vi "Test Basic Comm.vi"() -> ()   [LabVIEW 2011, in "Diamond Universal Driver.lvlib"]
uses:
  Diamond Universal Driver.lvlib
  Controls/board type.ctl
  Controls/dscBool.ctl
  Controls/dsccb.ctl
  constants.vi
  Controls/dscADSettings.ctl
  Controls/dscAIOint.ctl
  IO/DSCS.ctl
  Controls/gain.ctl
panel:
  out "data value":i16[](array[numeric])
  out "dscaioint 2":T1 {"ch_align" items=["FALSE", "TRUE"]; "fifo en" items=["FALSE", "TRUE"]; "int clk gate" items=["FALSE", "TRUE"]; "ext gate en" items=["FALSE", "TRUE"]; "intclk" items=["FALSE", "TRUE"]; "cycle" items=["FALSE", "TRUE"]}
  out "status":T3 {"analog" items=["FALSE", "TRUE"]}
  out "adSettingsOut":T4
  out "error out":errorcluster
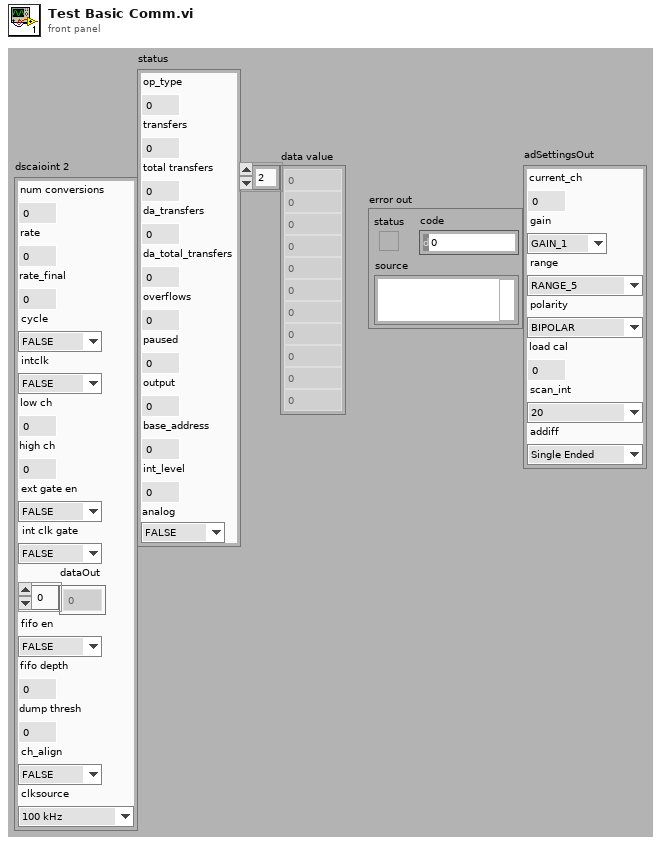
[diagram p1: front panel]
types:
  T1 = typedef "Diamond Universal Driver.lvlib/dscAIOint.ctl" = cluster{"num conversions":u32, "rate":sgl, "rate_final":sgl, "cycle":T2, "intclk":T2, "low ch":u8, "high ch":u8, "ext gate en":T2, "int clk gate":T2, "dataOut":i16[], "fifo en":T2, "fifo depth":u16, "dump thresh":u32, "ch_align":T2, "clksource":enum8{"100 kHz", "1 MHz"}}
  T2 = typedef "dscBool.ctl" = i32
  T3 = typedef "Diamond Universal Driver.lvlib/DSCS.ctl" = cluster{"op_type":u8, "transfers":u32, "total transfers":u32, "da_transfers":u32, "da_total_transfers":u32, "overflows":u32, "paused":u8, "output":u8, "base_address":u16, "int_level":u8, "analog":T2}
  T4 = typedef "dscADSettings.ctl" = cluster{"current_ch":u8, "gain":T5, "range":enum8{"RANGE_5", "RANGE_10"}, "polarity":enum16{"BIPOLAR", "UNIPOLAR"}, "load cal":u8, "scan_int":enum8{"20", "15", "10", "5", "9", "4"}, "addiff":enum8{"Single Ended", "Differential"}}
  T5 = typedef "gain.ctl" = enum8{"GAIN_1", "GAIN_2", "GAIN_8"}
  T6 = typedef "board type.ctl" = u8
  T7 = typedef "dsccb.ctl" = cluster{"board type":T6, "board num":i16, "base addr":u16, "int level":u8, "RMM external trig":T2, "RMM external trig c3":T2, "EMM IOAdd":u16[], "EMM IOInterrupt":u16[], "clkfreq0":enum8{"10 MHz", "1 MHz"}, "clkfreq1":enum8{"10 MHz", "1 MHz"}, "clksel1":enum8{"Internal (clkfrq1)", "External"}, "address space":dbl, "DAC cfg":u8, "clck_freq":i32, "dma_level":u8, "int_lvl 1":u8, "int_lvl 2":u8, "int_lvl 3":u8, "fpga":u16, "smm_ad_res":u8, "RMM mode 16bit":T2, "RMM DAC 0_3 ext en":T2, "RMM DAC 4_7 ext en":T2}
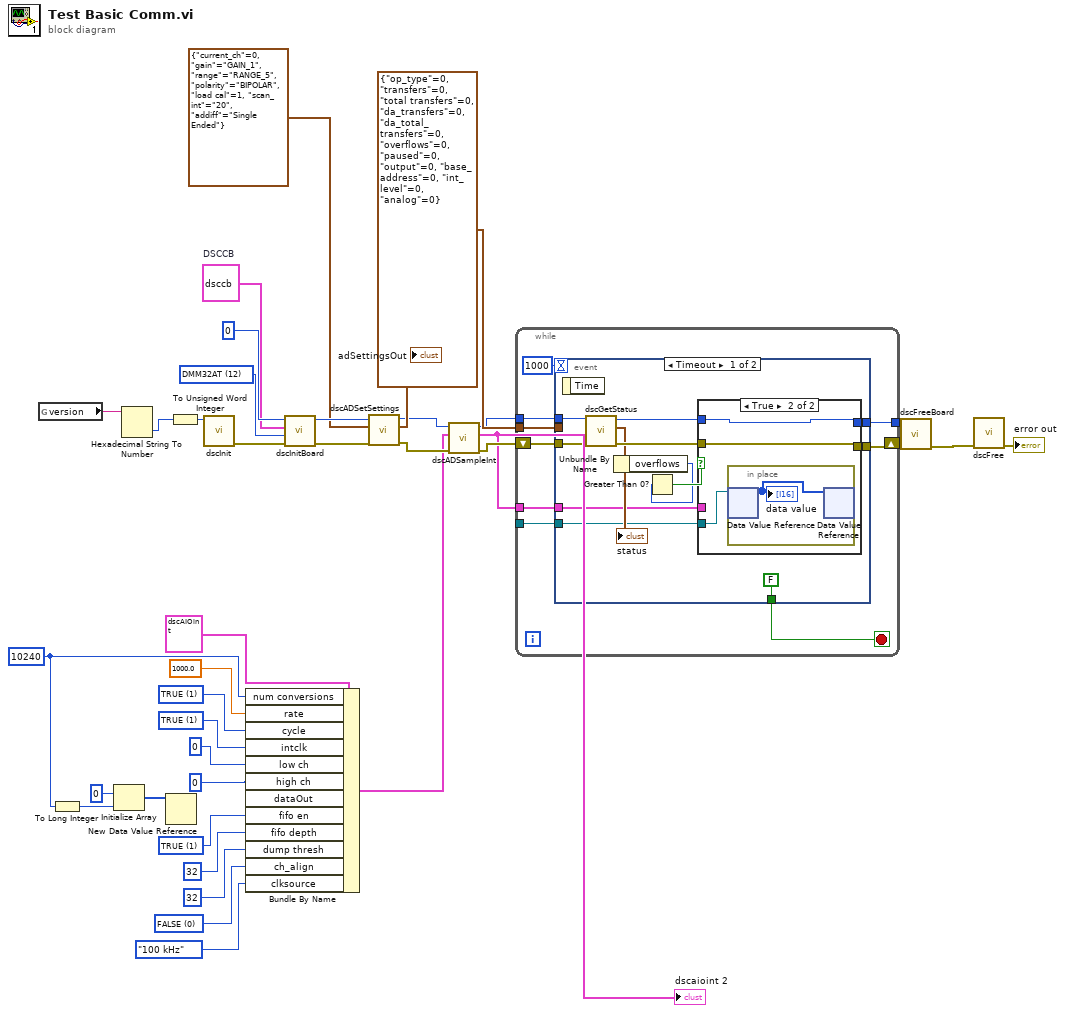
[diagram p0: block diagram]
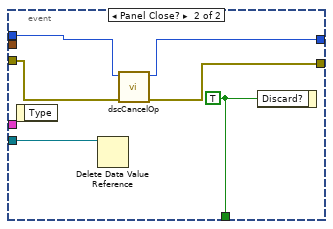
[diagram p3: hidden frame]
diagram:
  w4 = T2 0 items=["FALSE", "TRUE"] ("ch_align")
  w8 = T2 1 items=["FALSE", "TRUE"] ("fifo en")
  w13 = T2 1 items=["FALSE", "TRUE"] ("intclk")
  w14 = T2 1 items=["FALSE", "TRUE"] ("cycle")
  w10 = u32 10240 ("num conversions")
  w33 = T6 12 items=["DMM16"=0, "RMM"=1, "TMM"=2, "OPMM"=3, "DMM"=4, "SMM"=5, "GMM"=6, "QMM"=7, "ZMM"=8, "PMM"=9, "OMM"=10, "RMM416"=11, "DMM32AT"=12, "EMMDIO"=13, "RMM1612"=14, "DMMAT"=15, "DMM16AT"=16, "IR104"=17, "EMM8"=18, "PROM"=19, "HERCEBX"=20, "CPT"=21, "DMM48AT"=22, "OMMIO"=23, "DIO82C55"=24, "ATHENA"=25, "METIS"=26, "DMM32XAT"=27, "ELEKTRA"=28, "GPIO11_9513"=29, "GPIO11_DIO"=30, "GPIO21"=31, "PSD"=32, "ATHENAII"=33, "DMM32DXAT"=34, "HELIOS"=35, "NEPTUNE"=36, "TEST"=126, "RAW"=127, "DRVR"=255] ("board type")
  w29 = T7 {"board type"=12, "board num"=1, "base addr"=768, "int level"=3, "RMM external trig"=0, "RMM external trig c3"=0, "EMM IOAdd"=[0, 0, 0, 0, 0, 0, 0, 0], "EMM IOInterrupt"=[0, 0, 0, 0, 0, 0, 0, 0], "clkfreq0"=enum."10 MHz", "clkfreq1"=enum."10 MHz", "clksel1"=enum."Internal (clkfrq1)", "address space"=0.0, "DAC cfg"=0, "clck_freq"=0, "dma_level"=0, "int_lvl 1"=0, "int_lvl 2"=0, "int_lvl 3"=0, "fpga"=0, "smm_ad_res"=0, "RMM mode 16bit"=0, "RMM DAC 0_3 ext en"=0, "RMM DAC 4_7 ext en"=0}  # DSCCB
  n1 = global read "constants.vi" "version"() -> (w37:string)
  n2 = To Long Integer(number=w10) -> (32bit integer=w19:i32)
  n3 = Initialize Array(i16 0 ("element"), w19) -> (w17:i16[])
  n4 = Hexadecimal String To Number(string=w37) -> (number=w35:u32)  [unwired: 2 in, 1 out]
  n5 = New Data Value Reference(data value=w17) -> ()  [unwired: 1 in, 2 out]
  n6 = To Unsigned Word Integer(number=w35) -> (unsigned 16bit integer=w36:u16)
  n7 = call "dscInit.vi"("versionIn"=w36) -> ("error out"=w34:errorcluster)  [unwired: 9 in, 1 out]
  n8 = Bundle By Name(cluster=T1 {"num conversions"=0, "rate"=0.0, "rate_final"=0.0, "cycle"=0, "intclk"=0, "low ch"=0, "high ch"=0, "ext gate en"=0, "int clk gate"=0, "dataOut"=[], "fifo en"=0, "fifo depth"=0, "dump thresh"=0, "ch_align"=0, "clksource"=enum."100 kHz"} ("dscAIOint"), "num conversions"=w10, "rate"=sgl 1000.0, "cycle"=w14, "intclk"=w13, "low ch"=u8 0, "high ch"=u8 0, "fifo en"=w8, "fifo depth"=u16 32, "dump thresh"=u32 32, "ch_align"=w4, "clksource"=enum8{"100 kHz", "1 MHz"}."100 kHz") -> (w9:T1)  [unwired: 1 in]
  n9 = call "dscInitBoard.vi"("error in"=w34, "board type"=w33, "DSCCB"=w29, 11:u16 0 ("boardHandle")) -> ("error out"=w32:errorcluster, "boardHandleOut"=w30:i16)  [unwired: 5 in, 1 out]
  n10 = call "dscADSetSettings.vi"("error in"=w32, "adSettingsIn"=T4 {"current_ch"=0, "gain"=enum."GAIN_1", "range"=enum."RANGE_5", "polarity"=enum."BIPOLAR", "load cal"=1, "scan_int"=enum."20", "addiff"=enum."Single Ended"}, "boardIn"=w30) -> ("error out"=w18:errorcluster, "adSettingsOut"=→"adSettingsOut":T4, "boardOut"=w24:i16)  [unwired: 6 in]
  n11 = call "dscADSampleInt.vi"("error in"=w18, "dscAIOint"=w9, "boardIn"=w24) -> ("error out"=w22:errorcluster, "dscaioint"=w3:T1, "boardOut"=w23:i16)  [unwired: 6 in]
  "dscaioint 2" <- w3
  n12 = while {
    tunnel: w23 -> [w44]
    tunnel: T3 {"op_type"=0, "transfers"=0, "total transfers"=0, "da_transfers"=0, "da_total_transfers"=0, "overflows"=0, "paused"=0, "output"=0, "base_address"=0, "int_level"=0, "analog"=0} ("dscs") -> [w43]
    tunnel: [w42] -> w25
    shift-right: [w40] -> w21
    shift-left: w22 -> [w41]
    tunnel: _ -> [w39]
    tunnel: w3 -> [w38]
    stop <- w45 stop-if-true
    n13 = event shown="[0] Timeout" {
      selector: _ -> [_ _]
      dyn-events: _ -> [_ _]
      timeout: 1000 -> [_ _]
      tunnel: [FALSE ("Discard?") w70] -> w45
      tunnel: w44 -> [w57 w69]
      tunnel: w43 -> [_ _]
      tunnel: [w55 w68] -> w42
      tunnel: w41 -> [w54 w67]
      tunnel: [w52 w66] -> w40
      tunnel: w39 -> [w48 w65]
      tunnel: w38 -> [w47 _]
      event Timeout {
        n14 = event-data() -> ()  [unwired: 1 in, 1 out]
        n15 = call "dscGetStatus.vi"("error in"=w54, "board"=w57) -> ("error out"=w53:errorcluster, "status"=w51:T3, "boardOut"=w56:i16)  [unwired: 7 in]
        "status" <- w51
        n16 = Unbundle By Name(w51) -> ("overflows"=w49:u32)
        n17 = Greater Than 0?(x=w49) -> (x > 0?=w50:bool)
        n18 = case shown="True" w50 {
          tunnel: w56 -> [w60 w61]
          tunnel: [w60 w61] -> w55
          tunnel: w53 -> [w59 w62]
          tunnel: [w59 w62] -> w52
          tunnel: w48 -> [_ w63]
          tunnel: w47 -> [_ _]
          frame False {
          }
          frame True {
            n19 = in-place {
              n20 = in-place-dvr #1(w63) -> (w64:i16[])  [unwired: 1 out]
              "data value" <- w64
              n21 = in-place-dvr #1(w64) -> ()  [unwired: 2 out]
            }
          }
        }
      }
      event Panel Close? {
        w70 = TRUE ("Discard?")
        n22 = event-data() -> ()  [unwired: 1 in, 1 out]
        n23 = Delete Data Value Reference(data value reference=w65) -> ()  [unwired: 1 in, 2 out]
        n24 = call "dscCancelOp.vi"("error in"=w67, "board"=w69) -> ("error out"=w66:errorcluster, "boardOut"=w68:i16)  [unwired: 8 in]
        n25 = event-data("Discard?"=w70) -> ()  [unwired: 1 in, 1 out]
      }
    }
  }
  n26 = call "dscFreeBoard.vi"("error in"=w21, "boardIn"=w25) -> ("error out"=w2:errorcluster)  [unwired: 8 in, 1 out]
  n27 = call "dscFree.vi"("error in"=w2) -> ("error out"=→"error out":errorcluster)  [unwired: 10 in]
